vi "CheckFirstPulseForNegative.vi"(11 "pulses in":dbl[](array[numeric])) -> (3 "pulses out":dbl[](array[numeric]))   [LabVIEW 2017, in "CmsVirtualChannel.lvlib"]
uses:
  <vilib>/addons/InsightCM/Devices/Shared/Cms/CmsVirtualChannel/CmsVirtualChannel.lvlib
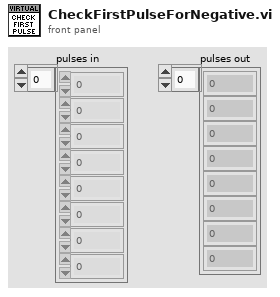
[diagram p1: front panel]
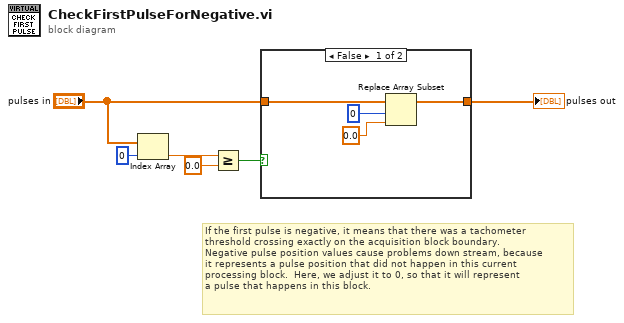
[diagram p0: block diagram]
diagram:
  # "If the first pulse is negative, it means that there was a tachometer\nthreshold crossing exactly on the acquisition block boundary.  \nNegative pulse position values cause problems down stream, because\nit represents a pulse position that did not happen in this current\nprocessing block.  Here, we adjust it to 0, so that it will represent\na pulse that happens in this block."
  n1 = Index Array(array="pulses in", index=0) -> (element=w5:dbl)
  n2 = Greater Or Equal?(x=w5, y=0.0) -> (x >= y?=w3:bool)
  n3 = case shown="False" w3 {
    tunnel: [w7 w11] -> w2
    tunnel: "pulses in" -> [w10 w11]
    frame False {
      n4 = Replace Array Subset(array=w10, new element=0.0 ("new element/subarray"), index=0) -> (w7:dbl[])
    }
    frame True {
    }
  }
  "pulses out" <- w2
